vi "K2200s_WaitKeyIccMeas2.vi"(8 "error Icc_In":errorcluster, 9 "VISA Icc_In":refnum<visa-resource-name>, 10 "Key":string, 11 "VISA Key_In":refnum<visa-resource-name>) -> (0 "error Icc_Out":errorcluster, 1 "VISA Icc_Out":refnum<visa-resource-name>, 3 "VISA Key_Out":refnum<visa-resource-name>, 5 "Icc, A":dbl, 7 "Icc, А":string)   [LabVIEW 2014]
uses:
  <vilib>/Utility/error.llb/whitespace.ctl
  C:/Users/rad/Desktop/Keithley 2200 Series Power Supplies Ver 1.2 (LV2009)/Keithley 2200 Series/Keithley 2200 Series.lvlib
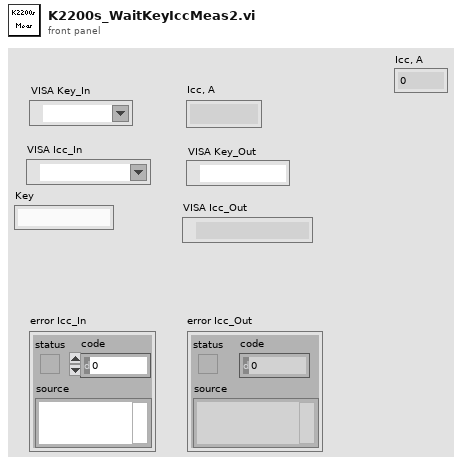
[diagram p1: front panel]
types:
  T1 = typedef "whitespace.ctl" = u16
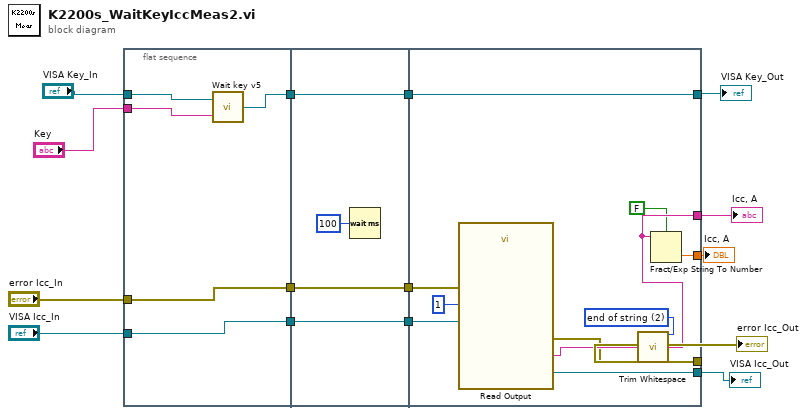
[diagram p0: block diagram]
diagram:
  n1 = flat-sequence {
    tunnel: [w20] -> w15
    tunnel: "VISA Key_In" -> [w19]
    tunnel: [w18] -> w14
    tunnel: "error Icc_In" -> [w18]
    tunnel: [w17] -> w13
    tunnel: "VISA Icc_In" -> [w17]
    tunnel: "Key" -> [w16]
    tunnel: w15 -> [w24]
    tunnel: [w24] -> w12
    tunnel: w14 -> [w23]
    tunnel: [w23] -> w11
    tunnel: w13 -> [w22]
    tunnel: [w22] -> w10
    tunnel: [w32] -> w5
    tunnel: w12 -> [w32]
    tunnel: w11 -> [w31]
    tunnel: w10 -> [w30]
    tunnel: [w29] -> w8
    tunnel: [w28] -> w9
    tunnel: [w27] -> w3
    tunnel: [w26] -> w2
    frame #0 {
      n2 = call "Wait key v5.vi"("Key"=w16, "VISA Refnum in"=w19) -> ("VISA Refnum out"=w20:refnum<visa-resource-name>)
    }
    frame #1 {
      n3 = Wait (ms)(milliseconds to wait=u32 100) -> ()  [unwired: 1 out]
    }
    frame #2 {
      w34 = T1 2 items=["both", "start of string", "end of string"] ("location (both)")
      n4 = call "Read Output.vi"("VISA resource name"=w30, "Measurement Function (0:Voltage)"=1, "error in (no error)"=w31) -> ("VISA resource name out"=w29:refnum<visa-resource-name>, "Measurement"=w33:string, "error out"=w28:errorcluster)  [unwired: 10 in]
      n5 = call <vilib>:"Trim Whitespace.vi"("string"=w33, "location (both)"=w34) -> ("trimmed string"=w27:string)
      n6 = Fract/Exp String To Number(use system decimal point (T)=FALSE, string=w27) -> (number=w26:dbl)  [unwired: 2 in, 1 out]
    }
  }
  "VISA Key_Out" <- w5
  "VISA Icc_Out" <- w8
  "error Icc_Out" <- w9
  "Icc, А" <- w3
  "Icc, A" <- w2
